vi "# + Comments +<EOL>.vi"(2 "Input String":string="This is a test\nit is a real test\nlet's see what is in\nthis box?\ntesting?\n", 3 "File Format":T1(ring)) -> (0 "Output String":string="This is a test\rit is a real test\rlet's see what is in\rthis box?\rtesting?\r")   [LabVIEW 2019]
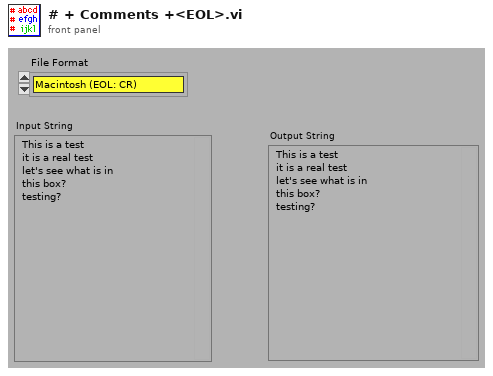
[diagram p1: front panel]
types:
  T1 = enum16{"Macintosh (EOL: CR)", "Unix (EOL: LF)", "DOS/Windows (EOL: CR+LF)"}
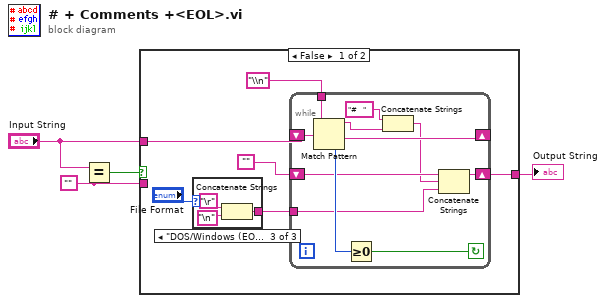
[diagram p0: block diagram]
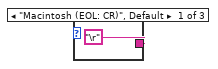
[diagram p2: hidden frame]
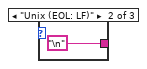
[diagram p3: hidden frame]
diagram:
  w1 = ""
  n1 = Equal?(x="Input String", y=w1) -> (x = y?=w3:bool)
  n2 = case shown="False" w3 {
    tunnel: "Input String" -> [w10 _]
    tunnel: [w9 w27] -> w4
    tunnel: w1 -> [_ w27]
    frame False {
      n3 = case shown="\"DOS/Windows (EOL: CR+LF)\"" "File Format" {
        tunnel: ["\r" "\n" w24] -> w5
        frame "Macintosh (EOL: CR)", Default {
        }
        frame "Unix (EOL: LF)" {
        }
        frame "DOS/Windows (EOL: CR+LF)" {
          n4 = Concatenate Strings("\r", "\n") -> (w24:string)
        }
      }
      n5 = while {
        tunnel: w5 -> [w11]
        shift-left: w10 -> [w19]
        shift-right: [w18] -> _
        shift-left: "" -> [w17]
        shift-right: [w16] -> w9
        tunnel: "\\n" -> [w21]
        stop <- w12 continue-if-true
        n6 = Match Pattern(string=w19, regular expression=w21) -> (before substring=w14:string, after substring=w18:string, offset past match=w20:i32)  [unwired: 1 in, 1 out]
        n7 = Greater Or Equal To 0?(x=w20) -> (x >= 0?=w12:bool)
        n8 = Concatenate Strings("#   ", w14) -> (w13:string)
        n9 = Concatenate Strings(w17, w13, w11) -> (w16:string)
      }
    }
    frame True {
    }
  }
  "Output String" <- w4
